vi "Configure Comparison Control.vi"(4 "Control Visibility":T2, 6 "Control Captions":T1, 7 "Control Refs":T3, 8 "error in (no error)":errorcluster) -> (0 "error out":errorcluster)   [LabVIEW 2016]
uses:
  Comparison Ctrl Refs.ctl
  Comparison Visibility.ctl
  Comparison Captions.ctl
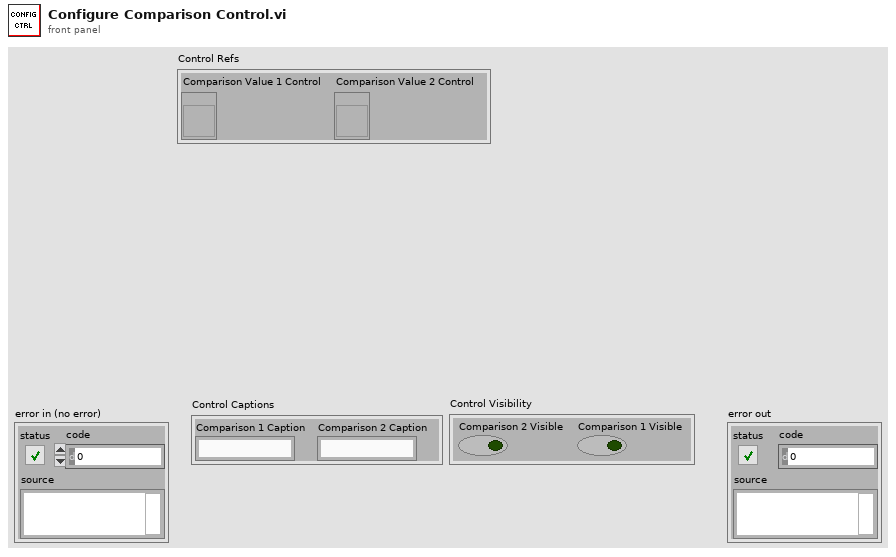
[diagram p1: front panel]
types:
  T1 = typedef "Comparison Captions.ctl" = cluster{"Comparison 1 Caption":string, "Comparison 2 Caption":string}
  T2 = typedef "Comparison Visibility.ctl" = cluster{"Comparison 2 Visible":bool, "Comparison 1 Visible":bool}
  T3 = typedef "Comparison Ctrl Refs.ctl" = cluster{"Comparison Value 1 Control":refnum<vi>, "Comparison Value 2 Control":refnum<vi>}
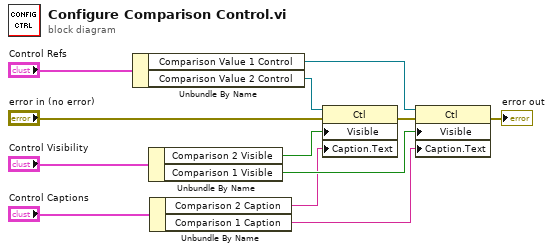
[diagram p0: block diagram]
diagram:
  n1 = Unbundle By Name("Control Refs") -> ("Comparison Value 1 Control"=w7:refnum<vi>, "Comparison Value 2 Control"=w8:refnum<vi>)
  n2 = Unbundle By Name("Control Visibility") -> ("Comparison 2 Visible"=w4:bool, "Comparison 1 Visible"=w3:bool)
  n3 = Unbundle By Name("Control Captions") -> ("Comparison 2 Caption"=w2:string, "Comparison 1 Caption"=w1:string)
  n4 = property class="Ctl"(reference=w8, error in="error in (no error)", "Visible"=w4, "Caption.Text"=w2) -> (error out=w11:errorcluster)  [unwired: 1 out]
  n5 = property class="Ctl"(reference=w7, error in=w11, "Visible"=w3, "Caption.Text"=w1) -> (error out=→"error out":errorcluster)  [unwired: 1 out]
